vi "selccionaGenerador.vi"(2 "error in (no error)":errorcluster) -> (0 "error out":errorcluster, 1 "Generador":string)   [LabVIEW 2019, in "AjustesPrevios.lvclass"]
uses:
  AjustesPrevios.lvclass
panel:
  in  "Interno":bool
  in  "Externo":bool
  # "Seleccione el tipo de generador"
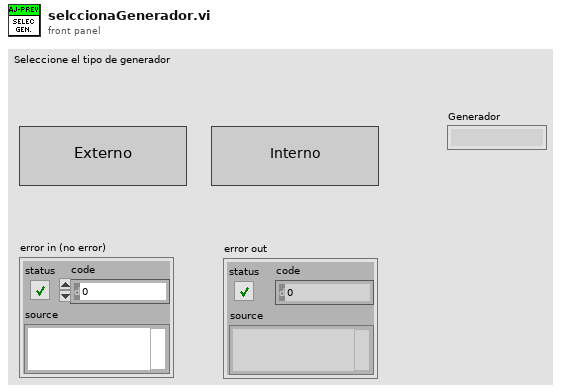
[diagram p1: front panel]
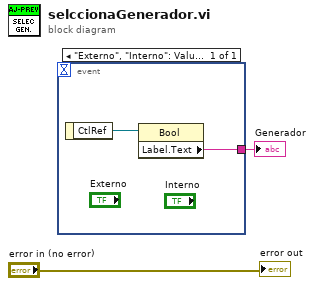
[diagram p0: block diagram]
diagram:
  n1 = event shown="[0] \"Externo\", \"Interno\": Value Change" {
    selector: _ -> [_]
    dyn-events: _ -> [_]
    timeout: _ -> [_]
    tunnel: [w3] -> w2
    event "Externo", "Interno": Value Change {
      n2 = event-data() -> ("CtlRef"=w4:refnum<vi>)  [unwired: 1 in]
      n3 = property class="Bool"(reference=w4) -> ("Label.Text"=w3:string)  [unwired: 1 in, 2 out]
    }
  }
  "Generador" <- w2
  "error out" <- "error in (no error)"
